vi "Control Path.vi"(11 "ElementEditorPanel in":refnum<class "ElementEditorPanel.lvclass">) -> (2 "Control Path":path)   [LabVIEW 2020, in "VolatusGUIControls.lvlib" / "ElementEditorPanel.lvclass"]
uses:
  ElementEditorPanel.lvclass
  ElementEditorPanel.lvclass/ElementEditorPanel.ctl
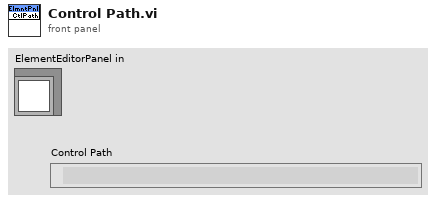
[diagram p1: front panel]
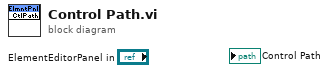
[diagram p0: block diagram]
diagram:
